vi "pMove_motor.vi"(8 "error in (no error)":errorcluster, 9 "mode (0: rel; 1: abs)":enum16{"relative", "absolute"}(ring), 10 "distance (pulses)":dbl, 11 "CCD in":refnum<class "Motor.lvclass">) -> (0 "error out":errorcluster, 3 "CCD out":refnum<class "Motor.lvclass">)   [LabVIEW 2016, in "Hardware.lvlib" / "Motor.lvlib" / "Motor.lvclass"]
doc: "move in position mode for the specified distance in the relative or absolute mode\n\nCopyright @ 2017 Fermion Instruments"
uses:
  <userlib>/Common Components/Hardware/Motor/Motor/Motor.lvclass
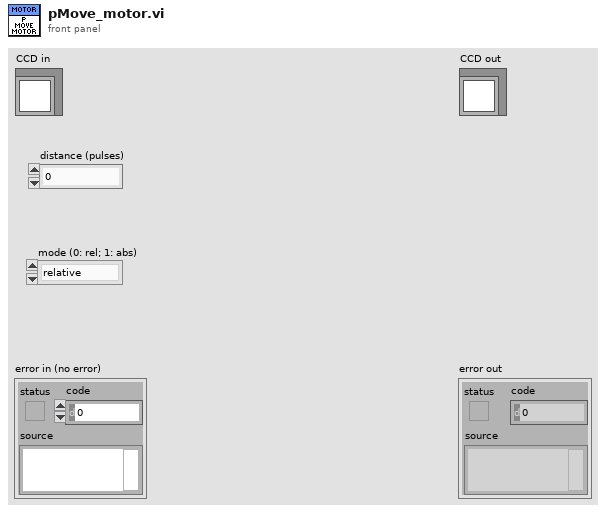
[diagram p1: front panel]
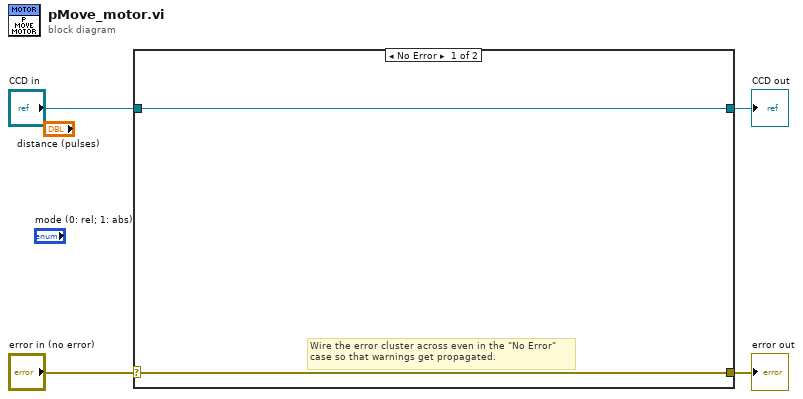
[diagram p0: block diagram]
diagram:
  n1 = case shown="No Error" "error in (no error)" {
    selector: "error in (no error)" -> [w5 w8]
    tunnel: [w5 w8] -> w3
    tunnel: [w6 w7] -> w1
    tunnel: "CCD in" -> [w6 w7]
    frame No Error {
      # "Wire the error cluster across even in the \"No Error\"\ncase so that warnings get propagated."
    }
    frame Error {
    }
  }
  "error out" <- w3
  "CCD out" <- w1
